vi "parameterized_SomeSessionsRegistered_InitializeAndCloseSessions_InitializeAndCloseCalledWithProperBehavior.vi"(0 "expected initialize-initialize calls":u32, 1 "initialize and close session behavior":T1, 5 "expected initialize-attach calls":u32, 7 "expected close-close calls":u32, 9 "expected close-detach calls":u32, 11 "error in":errorcluster) -> (4 "pass":bool, 6 "result":string, 15 "error out":errorcluster)   [LabVIEW 2020, in "MeasurementServerTests.lvlib"]
uses:
  MeasurementServerTests.lvlib
  Helpers/Fake Session Factory/Fake Session Factory.lvclass
  da6ffb6f-c1c9-4957-84dd-e9228483c454.vi
  ffc64c76-1568-41a3-8328-b9126ac9a28d.vi
  Runtime/APIs/Session Management V1/Session Reservation/Session Reservation.lvclass
  Runtime/APIs/Session Management V1/Session Reservation/Initialize and Close Session Behavior.ctl
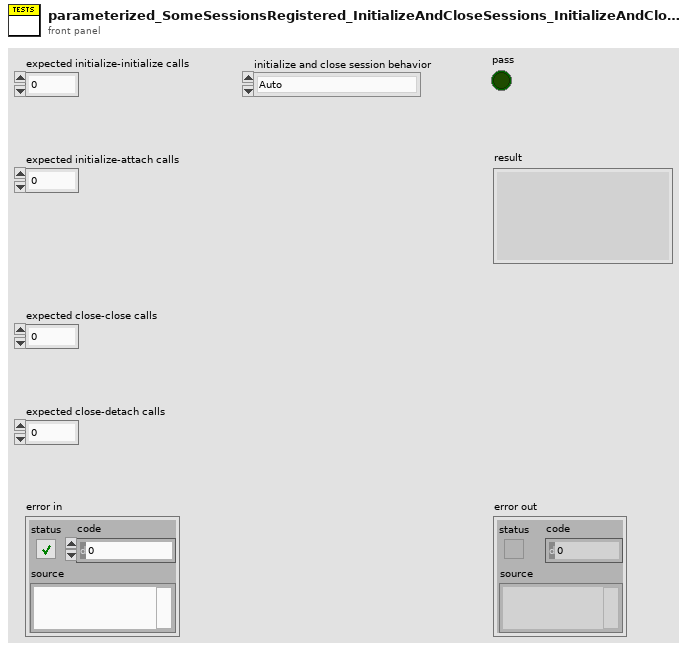
[diagram p1: front panel]
types:
  T1 = typedef "Plug-In SDK Session Management V1.lvlib/Session Reservation.lvclass/Initialize and Close Session Behavior.ctl" = enum16{"Auto", "Initialize and Close", "Attach and Detach", "Initialize and Detach", "Attach and Close"}
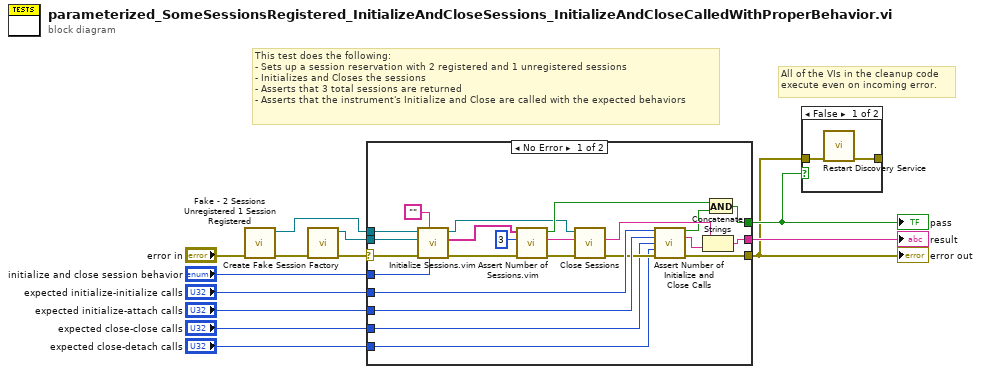
[diagram p0: block diagram]
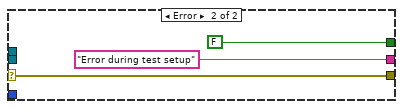
[diagram p2: hidden frame]
diagram:
  # "All of the VIs in the cleanup code\nexecute even on incoming error."
  # "This test does the following:\n- Sets up a session reservation with 2 registered and 1 unregistered sessions\n- Initializes and Closes the sessions\n- Asserts that 3 total sessions are returned\n- Asserts that the instrument's Initialize and Close are called with the expected behaviors"
  n1 = call "Fake - 2 Sessions Unregistered 1 Session Registered.vi"("error in"="error in") -> ("error out"=w7:errorcluster, "session reservation out"=w6:refnum<class "Session Reservation.lvclass">)  [unwired: 9 in]
  n2 = call "Create Fake Session Factory.vi"("error in"=w7) -> ("error out"=w10:errorcluster, "fake session factory out"=w9:refnum<class "Fake Session Factory.lvclass">)  [unwired: 9 in]
  n3 = case shown="No Error" w10 {
    selector: w10 -> [w33 w36]
    tunnel: [w26 w36] -> w11
    tunnel: [w25 FALSE] -> w12
    tunnel: [w23 "Error during test setup" ("f")] -> w13
    tunnel: w9 -> [w35 _]
    tunnel: w6 -> [w34 _]
    tunnel: "initialize and close session behavior" -> [w21 _]
    tunnel: "expected initialize-initialize calls" -> [w20 _]
    tunnel: "expected initialize-attach calls" -> [w19 _]
    tunnel: "expected close-close calls" -> [w15 _]
    tunnel: "expected close-detach calls" -> [w14 _]
    frame No Error {
      n4 = call "Initialize Sessions.vim"("initialize and close session behavior"=w21, "session type"="", "error in"=w33, "session factory"=w35, "session reservation in"=w34) -> ("error out"=w32:errorcluster, "sessions"=w30:string[], "session reservation out"=w16:refnum<class "Session Reservation.lvclass">)  [unwired: 3 in, 1 out]
      n5 = call "Assert Number of Sessions.vim"("error in"=w32, "expected number of sessions"=3, "sessions"=w30) -> ("error out"=w18:errorcluster, "result"=w29:string, "pass"=w28:bool)  [unwired: 6 in]
      n6 = call "Close Sessions.vi"("error in"=w18, "session reservation in"=w16) -> ("error out"=w17:errorcluster)  [unwired: 8 in, 1 out]
      n7 = call "Assert Number of Initialize and Close Calls.vi"("expected initialize-initialize calls"=w20, "expected initialize-attach calls"=w19, "expected close-close calls"=w15, "expected close-detach calls"=w14, "error in"=w17) -> ("pass"=w24:bool, "result"=w22:string, "error out"=w26:errorcluster)  [unwired: 8 in]
      n8 = Concatenate Strings(w29, w22) -> (w23:string)
      n9 = And(x=w28, y=w24) -> (x .and. y?=w25:bool)
    }
    frame Error {
    }
  }
  "error out" <- w11
  "pass" <- w12
  "result" <- w13
  n10 = case shown="False" w12 {
    tunnel: w11 -> [w40 _]
    tunnel: [w39 _] -> _
    frame False {
      n11 = call "Restart Discovery Service.vi"("error in"=w40) -> ("error out"=w39:errorcluster)  [unwired: 10 in]
    }
    frame True {
    }
  }
